vi "InputModeGet.vi"(0 "SR865 in":T2, 5 "error in":errorcluster) -> (14 "SR865 out":T2, 16 "InputMode":T1 caption="Input mode" items=["A", "A-B"], 19 "error out":errorcluster)   [LabVIEW 2017]
uses:
  SR865.ctl
  InputMode.ctl
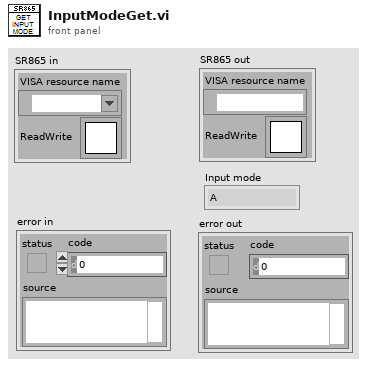
[diagram p1: front panel]
types:
  T1 = typedef "InputMode.ctl" = u16
  T2 = typedef "SR865.ctl" = cluster{"VISA resource name":refnum<visa-resource-name>, "ReadWrite":T3}
  T3 = typedef "Semaphore RefNum" = refnum<k1>
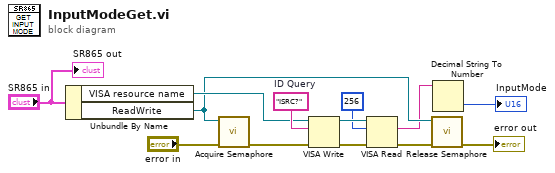
[diagram p0: block diagram]
diagram:
  w9 = "ISRC?"  # ID Query
  n1 = Unbundle By Name("SR865 in") -> ("VISA resource name"=w8:refnum<visa-resource-name>, "ReadWrite"=w3:T3)
  n2 = call <vilib>:"Acquire Semaphore.vi"("error in (no error)"="error in", "semaphore"=w3) -> ("error out"=w7:errorcluster)  [unwired: 3 in, 2 out]
  n3 = VISA Write(VISA resource name=w8, write buffer=w9, error in (no error)=w7) -> (VISA resource name out=w12:refnum<visa-resource-name>, error out=w11:errorcluster)  [unwired: 1 out]
  n4 = VISA Read(VISA resource name=w12, byte count=u32 256, error in (no error)=w11) -> (read buffer=w2:string, error out=w5:errorcluster)  [unwired: 2 out]
  n5 = call <vilib>:"Release Semaphore.vi"("error in (no error)"=w5, "semaphore"=w3) -> ("error out"=→"error out":errorcluster)  [unwired: 4 in, 1 out]
  n6 = Decimal String To Number(string=w2) -> (number=→"InputMode":i32)  [unwired: 2 in, 1 out]
  "SR865 out" <- "SR865 in"
